vi "Data_Array_Measurement.vi"(8 "error in (no error)":errorcluster, 10 "Measurement":dbl, 11 "Data_Array in":refnum<class "Data_Array.lvclass">) -> (0 "error out":errorcluster, 3 "Data_Array out":refnum<class "Data_Array.lvclass">)   [LabVIEW 2021, in "Data_Array.lvclass"]
uses:
  Data_Array.lvclass
  Data_Array.lvclass/Data_Array.ctl
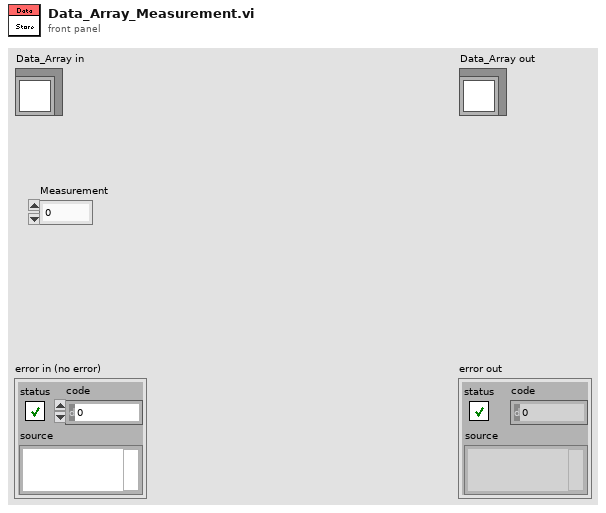
[diagram p1: front panel]
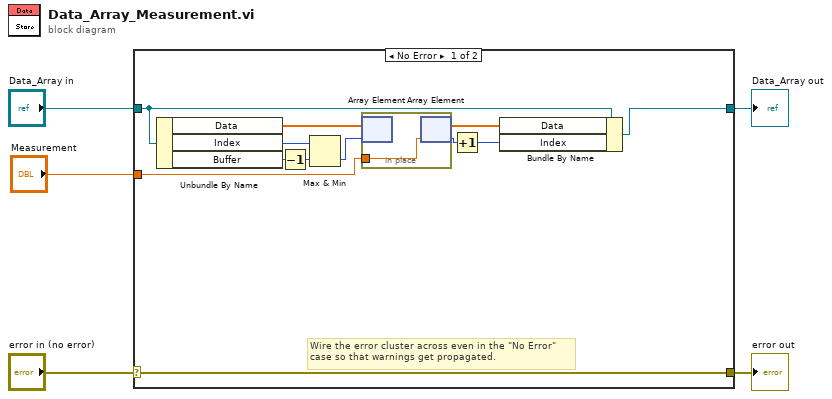
[diagram p0: block diagram]
diagram:
  n1 = case shown="No Error" "error in (no error)" {
    selector: "error in (no error)" -> [w17 w20]
    tunnel: [w17 w20] -> w4
    tunnel: [w6 w19] -> w2
    tunnel: "Data_Array in" -> [w9 w19]
    tunnel: "Measurement" -> [w12 _]
    frame No Error {
      # "Wire the error cluster across even in the \"No Error\"\ncase so that warnings get propagated."
      n2 = Unbundle By Name(w9) -> ("Data"=w16:dbl[], "Index"=w14:i32, "Buffer"=w13:i32)
      n3 = Decrement(x=w13) -> (x-1=w10:i32)
      n4 = Max & Min(x=w14, y=w10) -> (min(x,y)=w15:i32)  [unwired: 1 out]
      n5 = in-place {
        in-place-border: w12 -> [w18]
        n6 = in-place-array #1(w16, w15) -> ()  [unwired: 1 out]
        n7 = in-place-array #1(w18) -> (w7:dbl[], w11:i32)
      }
      n8 = Increment(x=w11) -> (x+1=w8:i32)
      n9 = Bundle By Name(cluster=w9, "Data"=w7, "Index"=w8) -> (w6:refnum<class "Data_Array.lvclass">)
    }
    frame Error {
    }
  }
  "error out" <- w4
  "Data_Array out" <- w2
